vi "Allocation RepCap.vi"(0 "Allocation In":T1=1, 1 "RepCap String In (\"\")":string) -> (2 "In Range?":bool, 3 "RepCap Identifier Out":string)   [LabVIEW 2020, in "Rohde&Schwarz CMXP NR FR2 Measurement.lvlib"]
doc: "Selects the Allocation repeated capability identifier for the selected Allocation value, and optionally appends it to the end of the repeated capability identifier string wired in to the RepCap String In terminal. The output string can be wired into the Repeated Capabilities terminal of the rscmxpnrfr2m ExpressVI."
uses:
  <instrlib>/Rohde&Schwarz CMXP NR FR2 Measurement/Rohde&Schwarz CMXP NR FR2 Measurement.lvlib
  <instrlib>/Rohde&Schwarz CMXP NR FR2 Measurement/Private/_Allocation.ctl
  <instrlib>/Rohde&Schwarz CMXP NR FR2 Measurement/Public/Utility/rsidr_core_global.vi
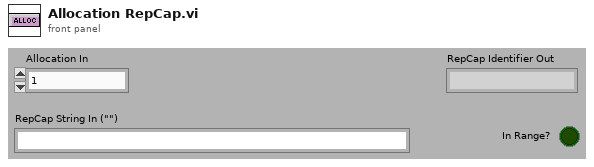
[diagram p1: front panel]
types:
  T1 = typedef "Rohde&Schwarz CMXP NR FR2 Measurement.lvlib/_Allocation.ctl" = i32
  T2 = cluster{"repCapName":string, "identifiers":string[], "cmdValues":string[]}[]
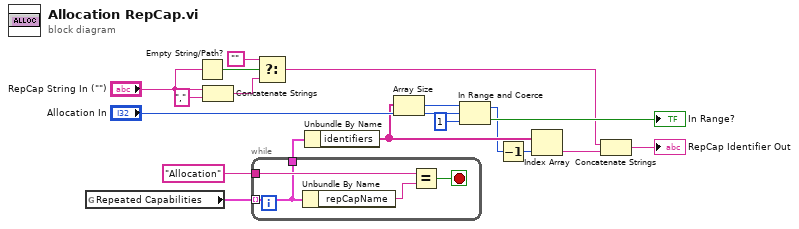
[diagram p0: block diagram]
diagram:
  n1 = global read "rsidr_core_global.vi" "Repeated Capabilities"() -> (w4:T2)
  n2 = Empty String/Path?(string/path="RepCap String In (\"\")") -> (empty?=w6:bool)
  n3 = Concatenate Strings("RepCap String In (\"\")", "," ("string")) -> (w9:string)
  n4 = while {
    tunnel: "Allocation" -> [w21]
    tunnel: w4 -> [w19] mode=indexing
    tunnel: [w19] -> w13
    stop <- w20 stop-if-true
    n5 = Unbundle By Name(w19) -> ("repCapName"=w22:string)
    n6 = Equal?(x=w21, y=w22) -> (x = y?=w20:bool)
  }
  n7 = Select(t="" ("Empty String Constant"), s=w6, f=w9) -> (s? t:f=w7:string)
  n8 = Unbundle By Name(w13) -> ("identifiers"=w16:string[])
  n9 = Array Size(array=w16) -> (size(s)=w1:i32)
  n10 = In Range and Coerce(upper limit=w1, x="Allocation In", lower limit=1) -> (coerced(x)=w3:T1, In Range?=→"In Range?":bool)
  n11 = Decrement(x=w3) -> (x-1=w2:T1)
  n12 = Index Array(array=w16, index=w2) -> (element=w11:string)
  n13 = Concatenate Strings(w7, w11) -> (→"RepCap Identifier Out":string)
